vi "N330X_Measure_Voltage.vi"(8 "error in (no error)":errorcluster, 11 "VISA Refnum in":refnum<visa-resource-name>) -> (0 "error out":errorcluster, 1 "Minimum Voltage":dbl, 2 "Total RMS Voltage":dbl, 3 "VISA Refnum out":refnum<visa-resource-name>, 4 "Maximum Voltage":dbl, 5 "Input Voltage":dbl)   [LabVIEW 2015]
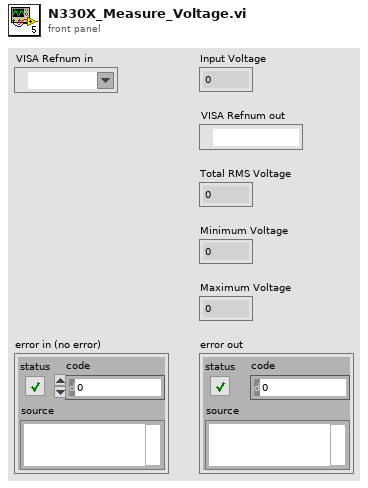
[diagram p1: front panel]
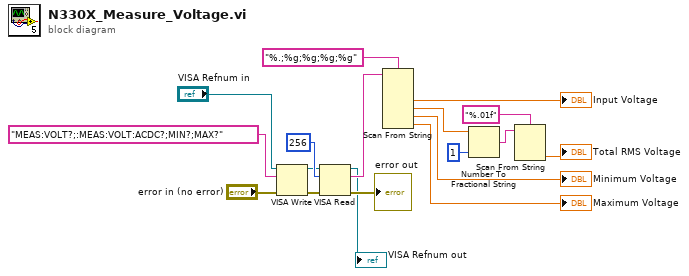
[diagram p0: block diagram]
diagram:
  n1 = VISA Write(VISA resource name="VISA Refnum in", write buffer="MEAS:VOLT?;:MEAS:VOLT:ACDC?;MIN?;MAX?", error in (no error)="error in (no error)") -> (VISA resource name out=w6:refnum<visa-resource-name>, error out=w8:errorcluster)  [unwired: 1 out]
  n2 = VISA Read(VISA resource name=w6, byte count=u32 256, error in (no error)=w8) -> (VISA resource name out=→"VISA Refnum out":refnum<visa-resource-name>, read buffer=w11:string, error out=→"error out":errorcluster)  [unwired: 1 out]
  n3 = Scan From String(format string="%.;%g;%g;%g;%g", input string=w11) -> (output 1=→"Input Voltage":dbl, output 2=w1:dbl, output 3=→"Minimum Voltage":dbl, output 4=→"Maximum Voltage":dbl)  [unwired: 6 in, 3 out]
  n4 = Number To Fractional String(number=w1, precision (6)=i16 1) -> (F-format string=w4:string)  [unwired: 2 in]
  n5 = Scan From String(format string="%.01f", input string=w4) -> (output 1=→"Total RMS Voltage":dbl)  [unwired: 3 in, 3 out]
